vi "set_N2.vi"(2 "Manifold N2 Flow":dbl, 3 "Display H2 or N2":bool, 4 "N2 Active":bool, 5 "H2N2 Remote":bool) -> ()   [LabVIEW 2011]
uses:
  editor_lib/Flow_Globals.vi
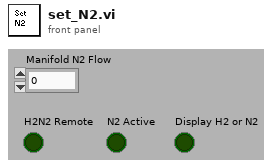
[diagram p1: front panel]
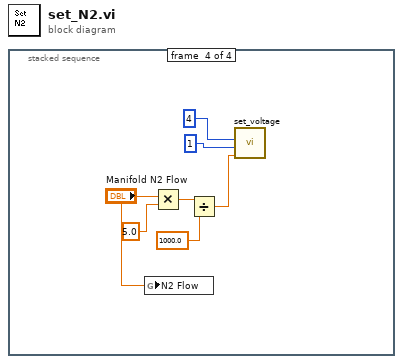
[diagram p0: block diagram]
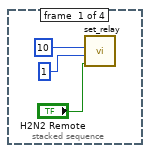
[diagram p2: hidden frame]
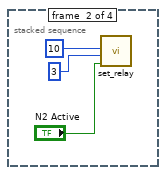
[diagram p3: hidden frame]
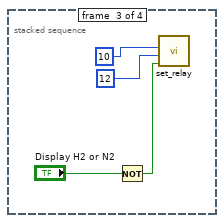
[diagram p4: hidden frame]
diagram:
  n1 = stacked-sequence {
    frame #0 {
      n2 = call "set_relay.vi"("Slot"=10, "Relay"=1, "Relay Status"="H2N2 Remote") -> ()  [unwired: 3 out]
    }
    frame #1 {
      n3 = call "set_relay.vi"("Slot"=10, "Relay"=3, "Relay Status"="N2 Active") -> ()  [unwired: 3 out]
    }
    frame #2 {
      n4 = Not(x="Display H2 or N2") -> (.not. x?=w10:bool)
      n5 = call "set_relay.vi"("Slot"=10, "Relay"=12, "Relay Status"=w10) -> ()  [unwired: 1 in, 2 out]
    }
    frame #3 {
      n6 = global write "Flow_Globals.vi" "N2 Flow"("Manifold N2 Flow") -> ()
      n7 = Multiply(x="Manifold N2 Flow", y=5.0) -> (x*y=w13:dbl)
      n8 = Divide(x=w13, y=1000.0) -> (x/y=w17:dbl)
      n9 = call "set_voltage.vi"("Voltage"=w17, "Channel"=1, "Slot"=4) -> ()  [unwired: 1 in, 1 out]
    }
  }
